vi "Radoslaw_Wolnik_3.2.vi"() -> ()   [LabVIEW 2020]
panel:
  in  "iloœæ generowanych liczb":i8
  in  "stop":bool
  out "Losowa liczba":i8
  # "Program generuje losow¹ liczbê w zakresie od 0 do 100 co 5s podan¹ iloœæ razy"
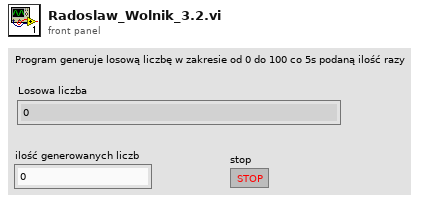
[diagram p1: front panel]
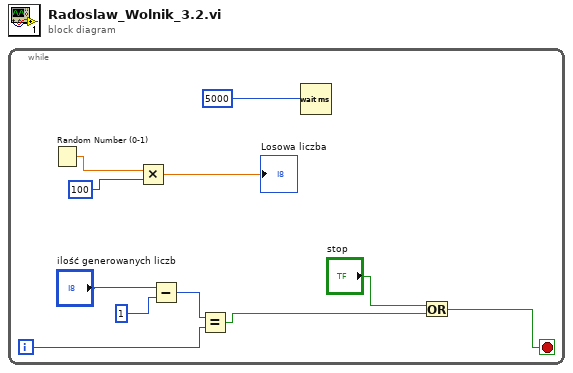
[diagram p0: block diagram]
diagram:
  n1 = while {
    i -> [w10]
    stop <- w7 stop-if-true
    n2 = Random Number (0-1)() -> (number: 0 to 1=w3:dbl)
    n3 = Multiply(x=w3, y=100) -> (x*y=→"Losowa liczba":dbl)
    n4 = Subtract(x="iloœæ generowanych liczb", y=1) -> (x-y=w6:i32)
    n5 = Equal?(x=w6, y=w10) -> (x = y?=w9:bool)
    n6 = Wait (ms)(milliseconds to wait=5000) -> ()  [unwired: 1 out]
    n7 = Or(x="stop", y=w9) -> (x .or. y?=w7:bool)
  }
